vi "Create and Sign JWT.vi"(6 "Additional Standard Claims":T1, 8 "error in (no error)":errorcluster, 9 "Key":string="@figbT|NKu|cn5P``Y!{gPpX3_e{bOe~", 10 "Signature Algorithm":T2, 11 "JSON Payload":string) -> (0 "error out":errorcluster, 2 "JWT":string, 3 "JWT out":refnum<class "JWT.lvclass">)   [LabVIEW 2020, in "JWT.lvlib" / "JWT.lvclass"]
uses:
  JWT.lvclass
  Signature Algorithms.ctl
  Additional Standard Claims.ctl
  JWT.lvclass/JWT.ctl
  lv-json/JSON/JSON.lvlib
  JWT.lvlib
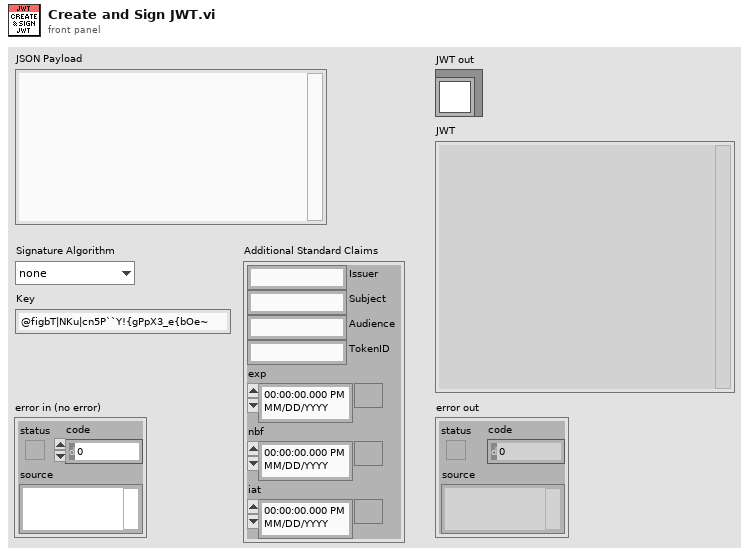
[diagram p1: front panel]
types:
  T1 = typedef "JWT.lvlib/JWT.lvclass/Additional Standard Claims.ctl" = cluster{"Issuer":string, "Subject":string, "Audience":string, "TokenID":string, "exp":timestamp, "nbf":timestamp, "iat":timestamp}
  T2 = typedef "JWT.lvlib/Signature Algorithms.ctl" = enum16{"none", "HS256"}
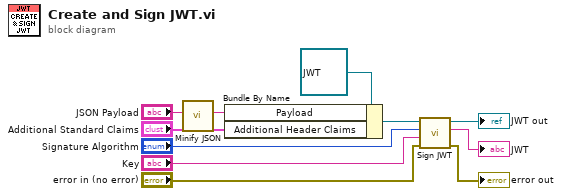
[diagram p0: block diagram]
diagram:
  n1 = call "Minify JSON.vi"("JSON String"="JSON Payload") -> ("Minified JSON"=w1:string)  [unwired: 10 in]
  n2 = Bundle By Name(cluster=refnum<class "JWT.lvclass"> refnum ("JWT out"), "Payload"=w1, "Additional Header Claims"="Additional Standard Claims") -> (w9:refnum<class "JWT.lvclass">)
  n3 = call "Sign JWT.vi"("error in (no error)"="error in (no error)", "Key"="Key", "Signature Algorithm"="Signature Algorithm", "JWT in"=w9) -> ("error out"=→"error out":errorcluster, "JWT"=→"JWT":string, "JWT out"=→"JWT out":refnum<class "JWT.lvclass">)  [unwired: 5 in]
